vi "LIN.vi"() -> ()   [LabVIEW 2015]
uses:
  <vilib>/xnet/xnet.llb/XNET Frame LIN.ctl
  <vilib>/xnet/xnet.llb/XNET Frame Type LIN.ctl
  <vilib>/xnet/xnet.llb/XNET LIN Diag Schedule Type.ctl
  <vilib>/xnet/xnet.llb/XNET Create Session (Frame Output Queued).vi
  <vilib>/xnet/xnet.llb/XNET Create Session (Frame Input Stream).vi
  <vilib>/xnet/xnet.llb/XNET Read (Frame LIN).vi
  <vilib>/xnet/xnet.llb/XNET Write (State LIN Diagnostic Schedule Change).vi
  <vilib>/xnet/xnet.llb/XNET Write (Frame LIN).vi
  <resource>/objmgr/xnet.rc
  <vilib>/xnet/xnet.llb/XNET Wait (Transmit Complete).vi
panel:
  out "data":T1[](array[typedef]) {"event ID" format="%x"; "payload" format="%x"; "timestamp" format="%<%.7X\n%x>T"; "type" items=["LIN Data"=64, "LIN Bus Error"=65, "LIN No Response"=66, "Delay"=224, "Log Trigger"=225, "Start Trigger"=226]; "identifier" format="%x"}
  in  "Frame Payloads to Queue":u8[][](array[numeric])=[[0, 0, 0, 0, 0, 0, 0, 0], [1, 1, 1, 1, 1, 1, 1, 1], [2, 2, 2, 2, 2, 2, 2, 2], [3, 3, 3, 3, 3, 3, 3, 3], [4, 4, 4, 4, 4, 4, 4, 4]]
  in  "Send":bool
  out "Frames":string[][](table)
  in  "Hex Display":bool
  in  "stop":bool
  in  "Number of Frames to Display":i32=15
  in  "interface":refnum<k21>="LIN1"
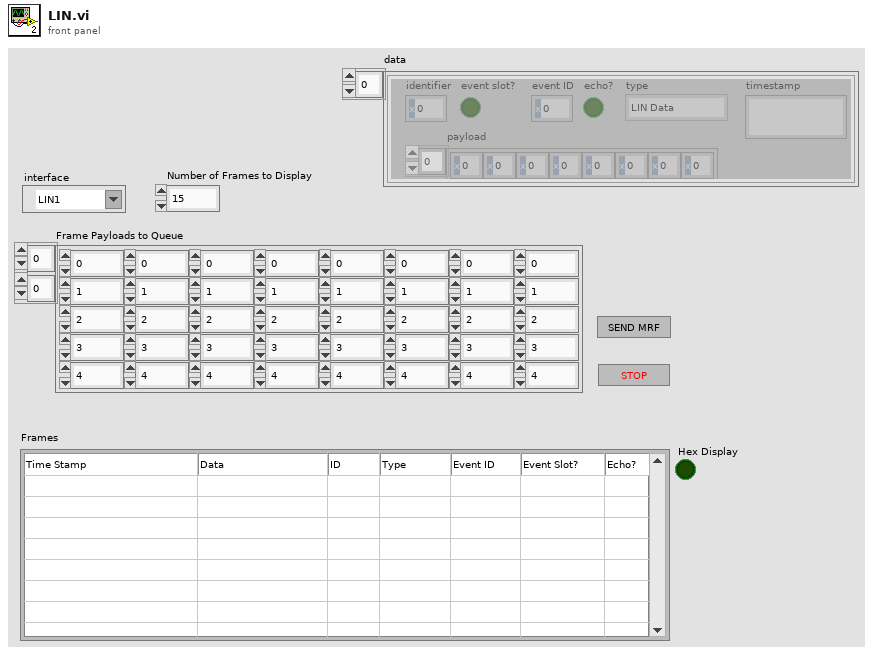
[diagram p1: front panel]
types:
  T1 = typedef "XNET Frame LIN.ctl" = cluster{"timestamp":timestamp, "payload":u8[], "identifier":u32, "type":T2, "event ID":u8, "event slot?":bool, "echo?":bool}
  T2 = typedef "XNET Frame Type LIN.ctl" = u8
  T3 = typedef "XNET LIN Diag Schedule Type.ctl" = u32
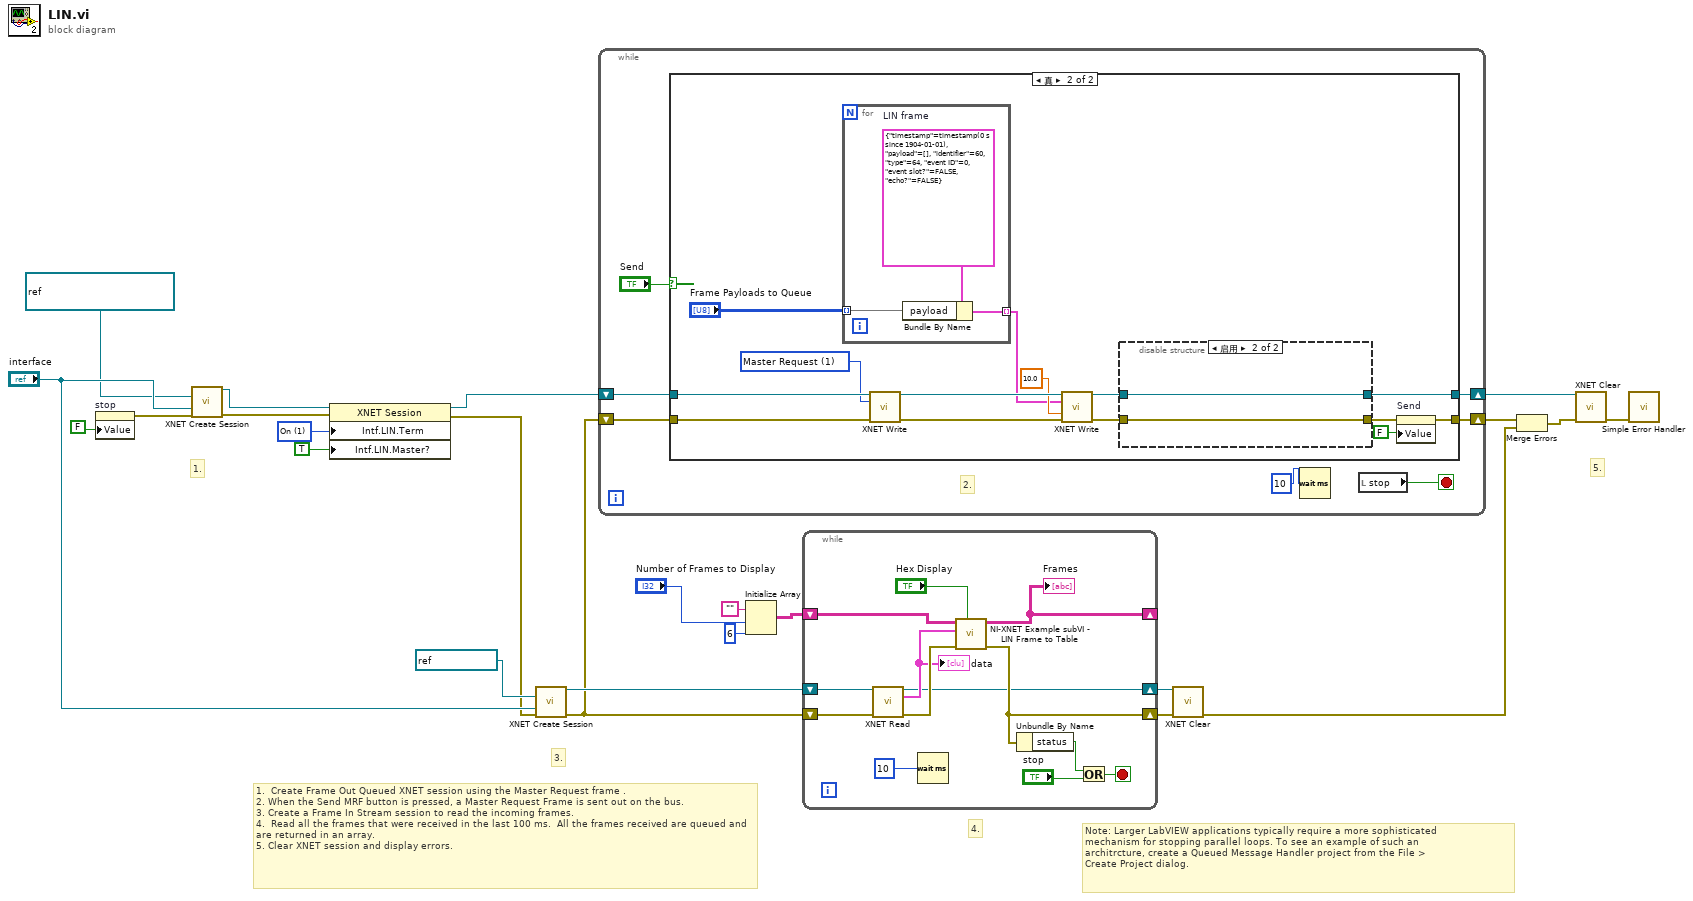
[diagram p0: block diagram]
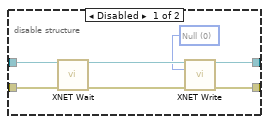
[diagram p3: hidden frame]
diagram:
  w22 = u32 1 items=["Off", "On"] ("Interface:LIN:Termination")
  # "5."
  # "4."
  # "3."
  # "1."
  # "1.  Create Frame Out Queued XNET session using the Master Request frame .\n2. When the Send MRF button is pressed, a Master Request Frame is sent out on the bus.\n3. Create a Frame In Stream session to read the incoming frames.\n4.  Read all the frames that were received in the last 100 ms.  All the frames received are queued and are returned in an array.  \n5. Clear XNET session and display errors."
  # "Note: Larger LabVIEW applications typically require a more sophisticated\nmechanism for stopping parallel loops. To see an example of such an \narchitrcture, create a Queued Message Handler project from the File >\nCreate Project dialog."
  n1 = property on="stop" class="Bool (严格)"("Value"=FALSE ("Send")) -> (error out=w1:errorcluster)  [unwired: 2 in, 1 out]
  n2 = call-poly <vilib>:"XNET Create Session.vi"("frame"=refnum<k21> "MasterReq\nNIXNET_exampleLDF", "interface"="interface", "error in (no error)"=w1) -> ("session out"=w23:refnum<k21>, "error out"=w24:errorcluster)  [unwired: 1 in, 10 out]
  n3 = property class="XNET Session"(reference=w23, error in=w24, "Intf.LIN.Term"=w22, "Intf.LIN.Master?"=TRUE ("Interface:LIN:Master?")) -> (reference out=w20:refnum<k21>, error out=w8:errorcluster)
  n4 = call-poly <vilib>:"XNET Create Session.vi"("cluster (:memory:)"=refnum<k21> ":memory:", "interface"="interface", "error in (no error)"=w8) -> ("session out"=w7:refnum<k21>, "error out"=w6:errorcluster)  [unwired: 11 out]
  n5 = while {
    shift-right: [w26] -> w5
    shift-left: w6 -> [w29]
    shift-right: [w30] -> w19
    shift-left: w20 -> [w31]
    stop <- w27 stop-if-true
    # "2."
    n6 = case shown="真" "Send" {
      tunnel: w31 -> [w33 w47]
      tunnel: [w33 w39] -> w30
      tunnel: w29 -> [w32 w37]
      tunnel: [w32 w35] -> w26
      frame False {
      }
      frame True {
        w44 = T3 1 items=["Null", "Master Request", "Slave Response"] ("diagnostics schedule (null)")
        n7 = for {
          tunnel: [w59] -> w40 mode=indexing
          tunnel: "Frame Payloads to Queue" -> [w57] mode=indexing
          w58 = T1 {"timestamp"=timestamp(0 s since 1904-01-01), "payload"=[], "identifier"=60, "type"=64, "event ID"=0, "event slot?"=FALSE, "echo?"=FALSE}  # LIN frame
          n8 = Bundle By Name(cluster=w58, "payload"=w57) -> (w59:T1)
        }
        n9 = call-poly <vilib>:"XNET Write.vi"("session in"=w47, "diagnostics schedule (null)"=w44, "error in (no error)"=w37) -> ("session out"=w46:refnum<k21>, "error out"=w45:errorcluster)  [unwired: 11 in]
        n10 = call-poly <vilib>:"XNET Write.vi"("session in"=w46, "data"=w40, "timeout (10)"=10.0, "error in (no error)"=w45) -> ("session out"=w42:refnum<k21>, "error out"=w41:errorcluster)  [unwired: 10 in]
        n11 = disable-structure shown="启用" {
          disable-tunnel: w42 -> [w54 w56]
          disable-tunnel: w41 -> [w53 w55]
          disable-tunnel: [w49 w56] -> w39
          disable-tunnel: [w48 w55] -> w36
          frame Disabled {
            w51 = T3 0 items=["Null", "Master Request", "Slave Response"] ("diagnostics schedule (null)")
            n12 = call-poly <vilib>:"XNET Wait.vi"("session in"=w54, "error in (no error)"=w53) -> ("session out"=w52:refnum<k21>, "error out"=w50:errorcluster)  [unwired: 12 in]
            n13 = call-poly <vilib>:"XNET Write.vi"("session in"=w52, "diagnostics schedule (null)"=w51, "error in (no error)"=w50) -> ("session out"=w49:refnum<k21>, "error out"=w48:errorcluster)  [unwired: 11 in]
          }
          frame Enabled {
          }
        }
        n14 = property on="Send" class="Bool (严格)"(error in=w36, "Value"=FALSE ("Send")) -> (error out=w35:errorcluster)  [unwired: 1 in, 1 out]
      }
    }
    n15 = Wait (ms)(milliseconds to wait=u32 10) -> ()  [unwired: 1 out]
    n16 = local read "stop"() -> (w27:bool)
  }
  n17 = Initialize Array("", "Number of Frames to Display", 6 ("Dimension Size")) -> (w15:string[][])
  n18 = while {
    shift-right: [w69] -> _
    shift-left: w15 -> [w70]
    shift-right: [w67] -> w12
    shift-left: w6 -> [w63]
    shift-right: [w64] -> w14
    shift-left: w7 -> [w62]
    stop <- w71 stop-if-true
    n19 = call-poly <vilib>:"XNET Read.vi"("session in"=w62, "error in (no error)"=w63) -> ("session out"=w64:refnum<k21>, "data"=w65:T1[], "error out"=w68:errorcluster)  [unwired: 11 out]
    "data" <- w65
    n20 = Wait (ms)(milliseconds to wait=u32 10) -> ()  [unwired: 1 out]
    n21 = call "NI-XNET Example subVI - LIN Frame to Table.vi"("Hexadecimal?"="Hex Display", "error in (no error)"=w68, "LIN Frames (from XNET Read)"=w65, "Input Array"=w70) -> ("error out"=w67:errorcluster, "Output Array"=w69:string[][])  [unwired: 1 in, 5 out]
    "Frames" <- w69
    n22 = Unbundle By Name(w67) -> ("status"=w72:bool)
    n23 = Or(x=w72, y="stop") -> (x .or. y?=w71:bool)
  }
  n24 = call <vilib>:"XNET Clear.vi"("session in"=w14, "error in (no error)"=w12) -> ("error out"=w4:errorcluster)  [unwired: 13 in]
  n25 = Merge Errors(w5, w4) -> (w3:errorcluster)
  n26 = call <vilib>:"XNET Clear.vi"("session in"=w19, "error in (no error)"=w3) -> ("error out"=w11:errorcluster)  [unwired: 13 out]
  n27 = call <vilib>:"Simple Error Handler.vi"("error in (no error)"=w11) -> ()  [unwired: 1 in, 8 out]
